vi "runTestScenario.vi"(8 "error in (no error)":errorcluster, 11 "ROT Test in":refnum<class "ROT Test.lvclass">) -> (0 "error out":errorcluster, 2 "TestExecution":T1, 3 "ROT Test out":refnum<class "ROT Test.lvclass">)   [LabVIEW 2015, in "ROT Test.lvclass"]
uses:
  ROT Test.lvclass
  Typedefs/TestExecution.ctl
  ROT Test.lvclass/ROT Test.ctl
  <userlib>/Common/ILC/ILC/ILC.lvclass/ILC.ctl
  Typedefs/WriteDataFileInput.ctl
  Typedefs/TestScenarioTypes.ctl
  Typedefs/WriteLogMessageInput.ctl
  Typedefs/PassFailTest.ctl
  Model/TestLog/ITestLog/ITestLog.lvclass
  Typedefs/ILCBTTypedefs.lvlib
  <userlib>/Common/ILC/ILC/ILC.lvclass
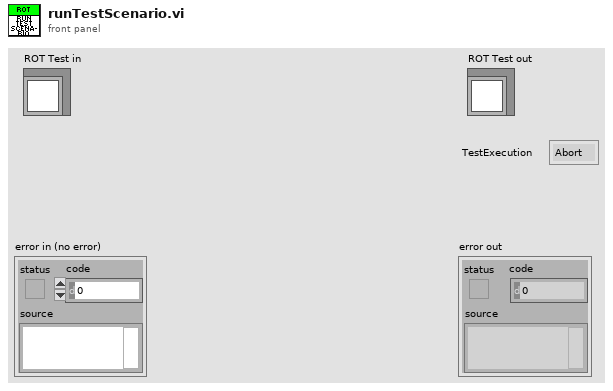
[diagram p1: front panel]
types:
  T1 = typedef "ILCBTTypedefs.lvlib/TestExecution.ctl" = enum16{"Abort", "Continue"}
  T2 = typedef "ILCBTTypedefs.lvlib/WriteLogMessageInput.ctl" = cluster{"Test Scenario":T3, "Description":string, "Actual Value":string, "Data File":string, "Result":T4}
  T3 = typedef "ILCBTTypedefs.lvlib/TestScenarioTypes.ctl" = enum16{"+3.3VA Supply Test", "+3.3VD Supply Test", "+5VA Supply Test", "+5VD Supply Test", "Unique ID Test", "TEDS Status Test", "LIMSW1_TTL Low Test", "LIMSW1_TTL High Test", "LIMSW2_TTL Low Test", "LIMSW2_TTL High Test", "Tachometer Test", "SSR_TTL Low Test", "SSR_TTL High Test", "SM_CW Low Test", "SM_CW High Test", "SM_CCW Low Test", "SM_CCW High Test", "SM_GPI Low Test", "SM_GPI High Test", "CW Motion Without Limit Test", "CW Motion With Limit Test", "CW Motion With Limit Interruption Test", "CW Motion on CCW Limit Test", "CCW Motion Without Limit Test", "CCW Motion With Limit Test", "CCW Motion With Limit Interruption Test", "CCW Motion on CW Limit Test", "RS232-TXD Low Test", "RS232-TXD High Test", "RS232-RTS Low Test", "RS232-RTS High Test", "RS232-RXD Low Test", "RS232-RXD High Test", "RS232-CTS Low Test", "RS232-CTS High Test", "Out_SS Low Test", "Out_SS High Test", "Out_SDI Low Test", "Out_SDI High Test", "Out_SCLK Low Test", "Out_SCLK High Test", "Reset Low Test", "Reset High Test", "1 Channel ADC Test", "3 Channel ADC Test", "5 Channel ADC Test", "Vref Test", "ROT Test", "DAC1 Test", "DAC2 Test", "DAC3 Test", "DAC4 Test", "BIAS Test", "EXC1 Test", "EXC2 Test", "EXC3 Test", "EXC4 Test"}
  T4 = typedef "ILCBTTypedefs.lvlib/PassFailTest.ctl" = enum16{"Fail", "Pass", "NA"}
  T5 = typedef "ILCBTTypedefs.lvlib/WriteDataFileInput.ctl" = cluster{"Test Scenario":T3, "File Name":string, "Output":dbl[]}
  T6 = typedef "ILCCommon.lvlib/ILCTypedefs.lvlib/OutputData.ctl" = cluster{"Step & Direction":i16, "Blower RPM":u8, "PWM (SSR)":u8, "Ch1":u16, "Ch2":u16, "Ch3":u16, "Ch4":u16}
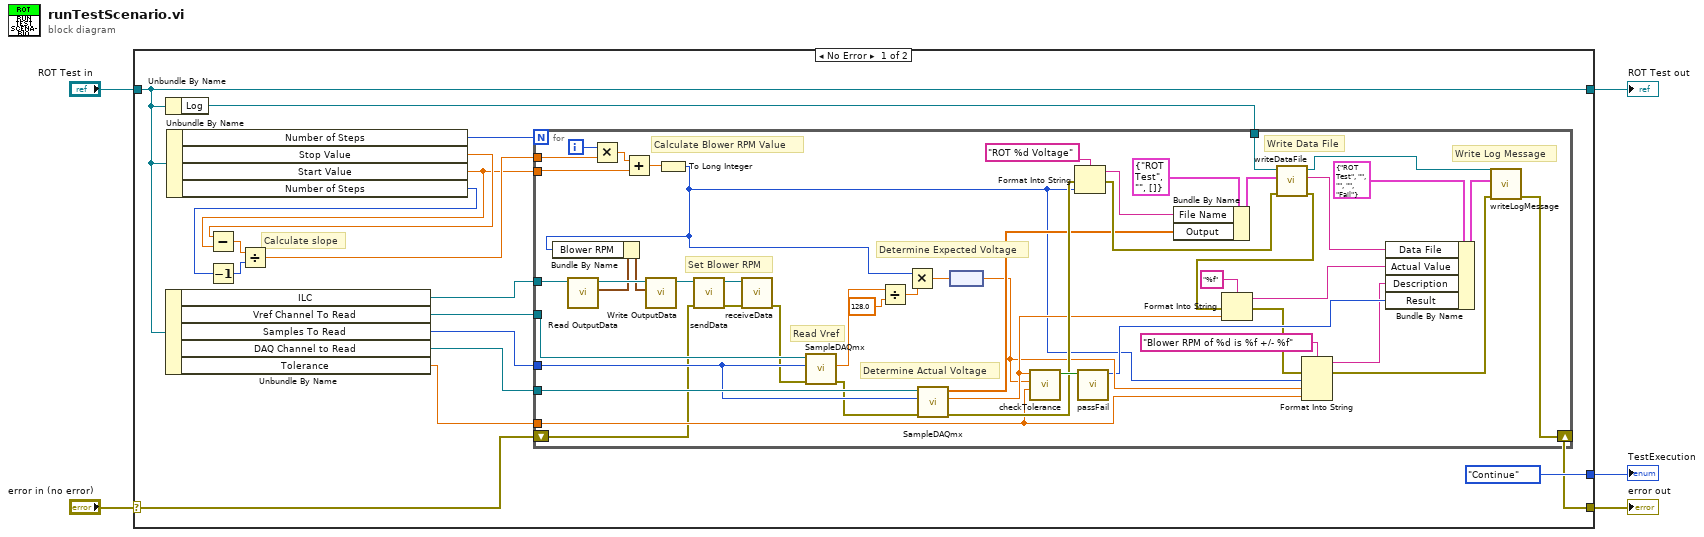
[diagram p0: block diagram]
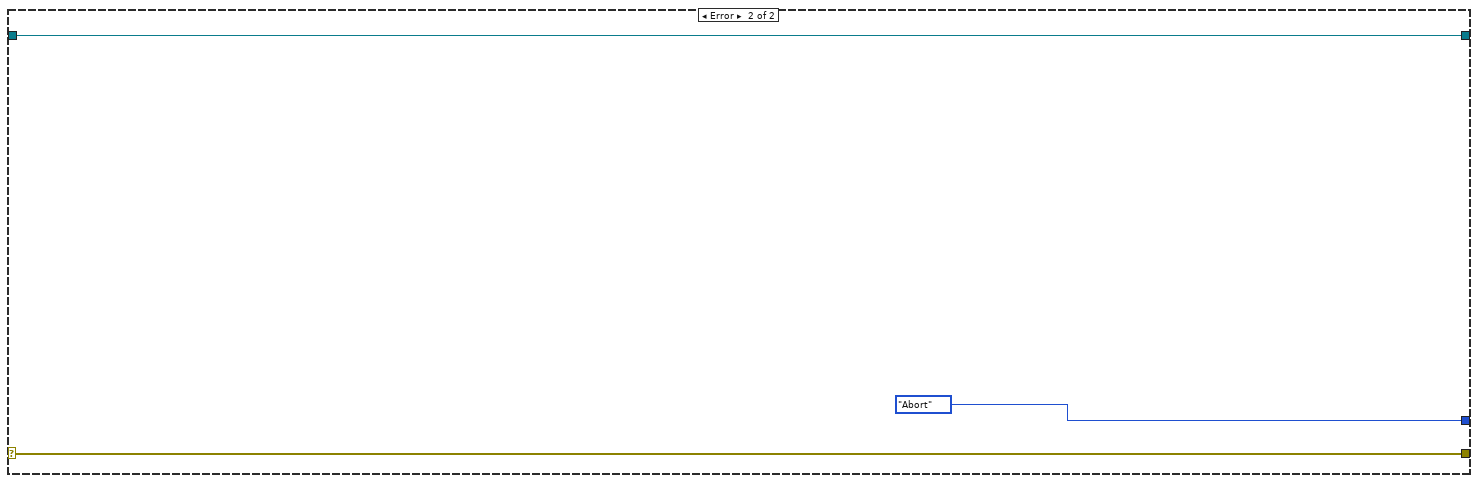
[diagram p2: hidden frame]
diagram:
  n1 = case shown="No Error" "error in (no error)" {
    selector: "error in (no error)" -> [w7 w73]
    tunnel: [w6 w73] -> w4
    tunnel: [TestExecution."Continue" ("TestExecution") TestExecution."Abort" ("TestExecution")] -> w3
    tunnel: "ROT Test in" -> [w9 w71]
    tunnel: [w9 w71] -> w1
    frame No Error {
      # "Calculate slope"
      n2 = Unbundle By Name(w9) -> ("Log"=w8:refnum<class "ITestLog.lvclass">)
      n3 = Unbundle By Name(w9) -> ("ILC"=w14:refnum<class "ILC.lvclass">, "Vref Channel To Read"=w13:refnum<k21>, "Samples To Read"=w12:i32, "DAQ Channel to Read"=w11:refnum<k21>, "Tolerance"=w10:dbl[unit])
      n4 = Unbundle By Name(w9) -> ("Number of Steps"=w15:u16, "Stop Value"=w21:dbl, "Start Value"=w16:dbl, "Number of Steps"=w18:u16)
      n5 = Subtract(x=w21, y=w16) -> (x-y=w20:dbl)
      n6 = Decrement(x=w18) -> (x-1=w19:u16)
      n7 = Divide(x=w20, y=w19) -> (x/y=w17:dbl)
      n8 = for {
        N: w15 -> [_]
        tunnel: w17 -> [w69]
        tunnel: w16 -> [w67]
        tunnel: w14 -> [w66]
        tunnel: w13 -> [w60]
        tunnel: w12 -> [w55]
        tunnel: w11 -> [w56]
        tunnel: w10 -> [w34]
        tunnel: w8 -> [w27]
        shift-right: [w26] -> w6
        shift-left: w7 -> [w25]
        i -> [w70]
        # "Write Log Message"
        # "Write Data File"
        # "Determine Actual Voltage"
        # "Set Blower RPM"
        # "Determine Expected Voltage"
        # "Read Vref"
        # "Calculate Blower RPM Value"
        n9 = call <userlib>:"Read OutputData.vi"("ILC in"=w66) -> ("OutputData"=w64:T6, "ILC out"=w65:refnum<class "ILC.lvclass">)  [unwired: 9 in]
        n10 = Multiply(x=w70, y=w69) -> (x*y=w68:dbl)
        n11 = Add(x=w68, y=w67) -> (x+y=w24:dbl)
        n12 = To Long Integer(number=w24) -> (32bit integer=w23:i32)
        n13 = Bundle By Name(cluster=w64, "Blower RPM"=w23) -> (w63:T6)
        n14 = call <userlib>:"Write OutputData.vi"("OutputData"=w63, "ILC in"=w65) -> ("ILC out"=w62:refnum<class "ILC.lvclass">)  [unwired: 9 in]
        n15 = call <userlib>:"sendData.vi"("error in (no error)"=w25, "ILC in"=w62) -> ("error out"=w48:errorcluster, "ILC out"=w61:refnum<class "ILC.lvclass">)  [unwired: 8 in]
        n16 = call <userlib>:"receiveData.vi"("error in (no error)"=w48, "ILC in"=w61) -> ("error out"=w49:errorcluster)  [unwired: 8 in, 1 out]
        n17 = call "SampleDAQmx.vi"("error in (no error)"=w49, "Samples To Read"=w55, "DAQ Channel To Read"=w60) -> ("error out"=w47:errorcluster, "Average"=w59:dbl)  [unwired: 6 in, 1 out]
        n18 = Divide(x=w59, y=128.0) -> (x/y=w57:dbl)
        n19 = Multiply(x=w23, y=w57) -> (x*y=w54:dbl)
        n20 = call "SampleDAQmx.vi"("error in (no error)"=w47, "Samples To Read"=w55, "DAQ Channel To Read"=w56) -> ("error out"=w46:errorcluster, "Average"=w38:dbl, "Samples"=w43:dbl[])  [unwired: 6 in]
        n21 = node(w54) -> (w33:dbl[unit])
        n22 = call "checkTolerance.vi"("Tolerance"=w34, "Expected Value"=w33, "Average"=w38) -> ("Boolean"=w53:bool)  [unwired: 8 in]
        n23 = Format Into String(format string="ROT %d Voltage", error in=w46, w23) -> (resulting string=w44:string, error out=w45:errorcluster)  [unwired: 1 in]
        n24 = call "passFail.vi"("Boolean"=w53) -> ("Result"=w32:T4)  [unwired: 10 in]
        n25 = Bundle By Name(cluster=T5 {"Test Scenario"=enum."ROT Test", "File Name"="", "Output"=[]} ("WriteDataFileInput"), "File Name"=w44, "Output"=w43) -> (w50:T5)
        n26 = call-dynamic "writeDataFile.vi"("error in (no error)"=w45, "WriteDataFileInput"=w50, "ITestLog in"=w27) -> ("error out"=w37:errorcluster, "Relative Path"=w40:string, "ITestLog out"=w42:refnum<class "ITestLog.lvclass">)  [unwired: 6 in]
        n27 = Format Into String(format string="%f", error in=w37, w38) -> (resulting string=w36:string, error out=w30:errorcluster)  [unwired: 1 in]
        n28 = Format Into String(format string="Blower RPM of %d is %f +/- %f", error in=w30, w23, w33, w34) -> (resulting string=w31:string, error out=w28:errorcluster)  [unwired: 1 in]
        n29 = Bundle By Name(cluster=T2 {"Test Scenario"=enum."ROT Test", "Description"="", "Actual Value"="", "Data File"="", "Result"=enum."Fail"} ("WriteLogMessageInput"), "Data File"=w40, "Actual Value"=w36, "Description"=w31, "Result"=w32) -> (w29:T2)
        n30 = call-dynamic "writeLogMessage.vi"("error in (no error)"=w28, "WriteLogMessageInput"=w29, "ITestLog in"=w42) -> ("error out"=w26:errorcluster)  [unwired: 7 in, 1 out]
      }
    }
    frame Error {
    }
  }
  "ROT Test out" <- w1
  "error out" <- w4
  "TestExecution" <- w3
